vi "Get DVR for class.vi"() -> ()   [LabVIEW 2020, in "Test.lvclass"]
uses:
  Test.lvclass
panel:
  in  "Error In":errorcluster
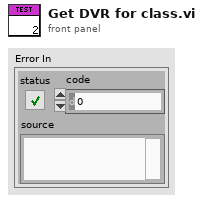
[diagram p1: front panel]
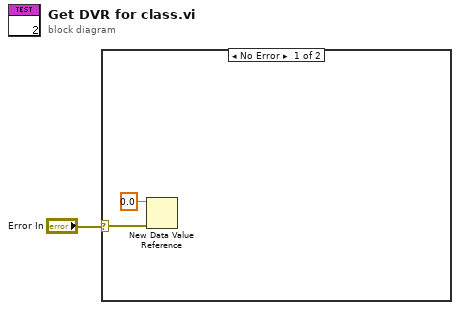
[diagram p0: block diagram]
diagram:
  n1 = case shown="No Error" "Error In" {
    selector: "Error In" -> [w3 _]
    frame No Error {
      n2 = New Data Value Reference(data value=0.0, error in=w3) -> ()  [unwired: 2 out]
    }
    frame Error {
    }
  }
